vi "getGenReadUserEvent.vi"(8 "error in (no error)":errorcluster, 11 "TcpServer in":refnum<class "TcpServer.lvclass">) -> (0 "error out":errorcluster, 2 "GenRead":refnum<user-event>, 3 "TcpServer out":refnum<class "TcpServer.lvclass">)   [LabVIEW 2018, in "TcpServerCmd.lvclass"]
doc: "Get the GenRead user event reference."
uses:
  TcpServerCmd.lvclass
  TcpServer/TcpServer.lvclass
  TcpServerBase/typedef/connStatusCluster.ctl
  TcpServer/TcpServer.lvclass/TcpServer.ctl
  TcpServerBase/TcpServerBase.lvclass/TcpServerBase.ctl
  home/pcortes/github/ts_labview_tcp_json/src/TcpServerBase/TcpServerBase.lvclass
  TcpServerBase/TcpServerBase.lvclass
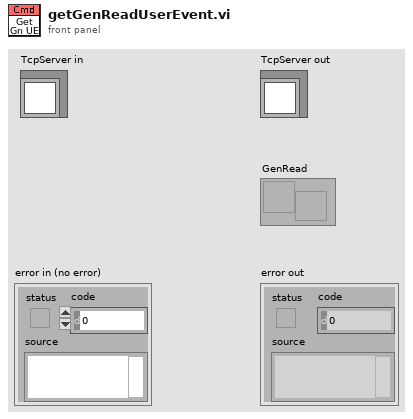
[diagram p1: front panel]
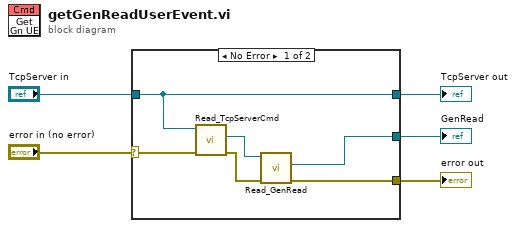
[diagram p0: block diagram]
diagram:
  n1 = case shown="No Error" "error in (no error)" {
    selector: "error in (no error)" -> [w9 w12]
    tunnel: "TcpServer in" -> [w6 w13]
    tunnel: [w8 w12] -> w3
    tunnel: [w7 _] -> w2
    tunnel: [w6 w13] -> w1
    frame No Error {
      n2 = call "Read_TcpServerCmd.vi"("error in (no error)"=w9, "TcpServer in"=w6) -> ("error out"=w10:errorcluster, "TcpServerCmd.lvclass"=w11:refnum<class "TcpServerCmd.lvclass">)  [unwired: 7 in, 1 out]
      n3 = call "Read_GenRead.vi"("error in (no error)"=w10, "TcpServerBase in"=w11) -> ("error out"=w8:errorcluster, "GenRead"=w7:refnum<user-event>)  [unwired: 7 in, 1 out]
    }
    frame Error {
    }
  }
  "TcpServer out" <- w1
  "error out" <- w3
  "GenRead" <- w2
